vi "forceIncludeZeroes.vi"(8 "forceX0":bool, 9 "forceY0":bool, 10 "XY Graph Cluster":cluster{dbl[], dbl[]}[](array[cluster]) {"?" format="%.2f"; "?" format="%.2f"}) -> (2 "appended array":cluster{"Array":dbl[], "Array":dbl[]}[](array[cluster]))   [LabVIEW 2020]
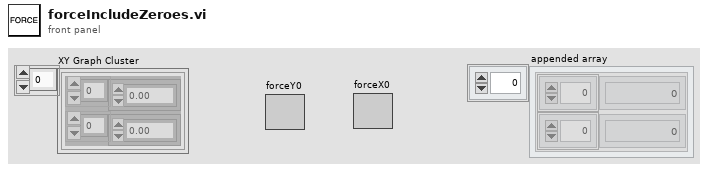
[diagram p1: front panel]
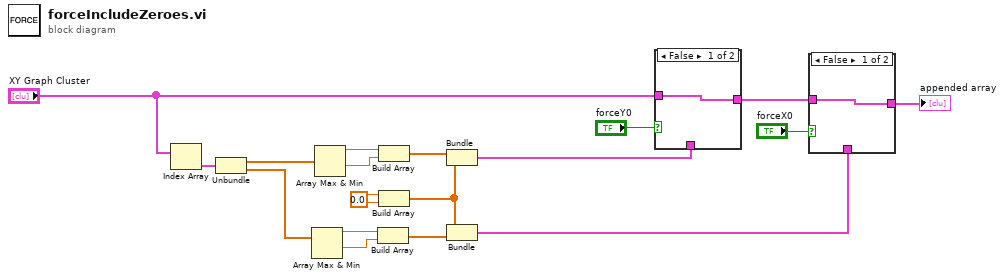
[diagram p0: block diagram]
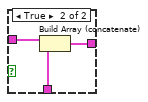
[diagram p2: hidden frame]
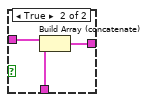
[diagram p3: hidden frame]
diagram:
  w14 = 0.0
  n1 = Index Array(array="XY Graph Cluster") -> (element=w18:cluster{dbl[], dbl[]})  [unwired: 1 in]
  n2 = Unbundle(w18) -> (w17:dbl[], w10:dbl[])
  n3 = Array Max & Min(array=w10) -> (max value=w11:dbl, min value=w12:dbl)  [unwired: 2 out]
  n4 = Array Max & Min(array=w17) -> (max value=w16:dbl, min value=w15:dbl)  [unwired: 2 out]
  n5 = Build Array(w11, w12) -> (w9:dbl[])
  n6 = Build Array(w16, w15) -> (w13:dbl[])
  n7 = Build Array(w14, w14) -> (w8:dbl[])
  n8 = Bundle(w13, w8) -> (w7:cluster{dbl[], dbl[]})  [unwired: 1 in]
  n9 = Bundle(w8, w9) -> (w2:cluster{dbl[], dbl[]})  [unwired: 1 in]
  n10 = case shown="False" "forceY0" {
    tunnel: "XY Graph Cluster" -> [w19 w22]
    tunnel: [w19 w21] -> w5
    tunnel: w7 -> [_ w20]
    frame False {
    }
    frame True {
      n11 = Build Array (concatenate)(w22, w20) -> (w21:cluster{dbl[], dbl[]}[])
    }
  }
  n12 = case shown="False" "forceX0" {
    tunnel: w5 -> [w23 w26]
    tunnel: [w23 w25] -> w4
    tunnel: w2 -> [_ w24]
    frame False {
    }
    frame True {
      n13 = Build Array (concatenate)(w26, w24) -> (w25:cluster{dbl[], dbl[]}[])
    }
  }
  "appended array" <- w4
